vi "OA_ConnectToOrigin.vi"(5 "Visible":i32(ring)=1 items=["MAINWND_HIDE"=0, "MAINWND_SHOW"=1, "MAINWND_SHOWMINIMIZED"=2, "MAINWND_SHOWMAXIMIZED"=3, "MAINWND_SHOW_BRING_TO_FRONT"=100], 6 "error in (no error)":errorcluster) -> (0 "error out":errorcluster, 3 "Origin.IOApplication":refnum<k7>)   [LabVIEW 2010]
doc: "Connect to Origin project and show the main window of Origin. Using ApplicationSI, and will not open new instance."
panel:
  in  "Origin.IOApplicationSI":refnum<k7>
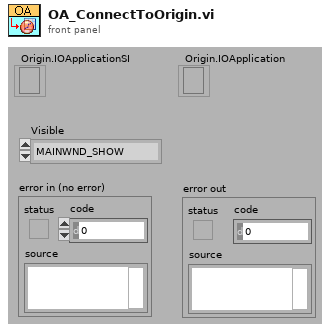
[diagram p1: front panel]
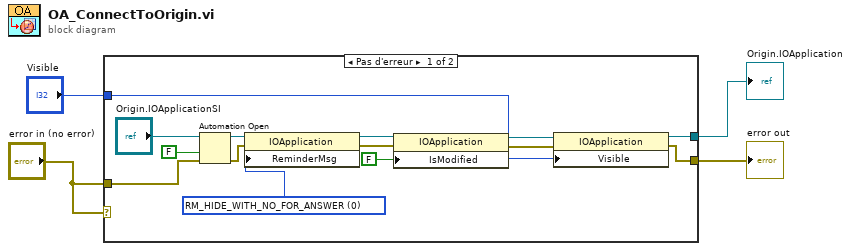
[diagram p0: block diagram]
diagram:
  n1 = case shown="Pas d'erreur" "error in (no error)" {
    tunnel: "error in (no error)" -> [w8 w19]
    tunnel: [w18 _] -> w4
    tunnel: [w17 w19] -> w3
    tunnel: "Visible" -> [w6 _]
    frame No Error {
      w16 = 0 items=["RM_LET_ORIGIN_DECIDE"=-1, "RM_HIDE_WITH_NO_FOR_ANSWER"=0, "RM_HIDE_WITH_YES_FOR_ANSWER"=1] ("ReminderMsg")
      n2 = Automation Open(error in (no error)=w8, Automation Refnum="Origin.IOApplicationSI", 9:FALSE ("open new instance")) -> (Automation Refnum=w10:refnum<k7>, error out=w11:errorcluster)  [unwired: 1 in]
      n3 = property class="IOApplication"(reference=w10, error in=w11, "ReminderMsg"=w16) -> (reference out=w15:refnum<k7>, error out=w13:errorcluster)
      n4 = property class="IOApplication"(reference=w15, error in=w13, "IsModified"=FALSE) -> (reference out=w14:refnum<k7>, error out=w12:errorcluster)
      n5 = property class="IOApplication"(reference=w14, error in=w12, "Visible"=w6) -> (reference out=w18:refnum<k7>, error out=w17:errorcluster)
    }
    frame Error {
    }
  }
  "Origin.IOApplication" <- w4
  "error out" <- w3
